vi "Configure.vi"(0 "Interface in":T5, 5 "Configuration":T1={"PLLgains"={"proportional gain"=0.0, "integral gain"=0.0}, "PLLrange"={"output high (Inf)"=inf, "output low (-Inf)"=-inf}, "dT"=0.0, "expectedFreq"=0.0, "lockDuration"=0.0, "freqBoundaries"=0.0, "adjustTheta"=0.0, "HarmonicFilter"={"enable"=FALSE, "coeff"={"ak"=0.0, "bk"=0.0}}} {"PLLgains"."proportional gain" step=0.125}, 11 "error in":errorcluster) -> (4 "Interface out":T5, 15 "error out":errorcluster)   [LabVIEW 2017, in "ThreePhasePLLInterface.lvlib"]
uses:
  ThreePhasePLLInterface.lvlib
  InterfaceRef.ctl
  <instrlib>/_niInstr/Instruction Framework/v1/Host/Instruction Target/niInstr Instruction Target v1 Host.lvclass
  <instrlib>/_niInstr/Instruction Framework/v1/Host/Instruction Framework Context/niInstr Instruction Framework Context v1 Host.lvclass
  Configuration.ctl
  <vilib>/rvi/Analysis/control/PID/Typedef/niFpgaPID_PIGains.ctl
  <vilib>/rvi/Analysis/control/PID/Typedef/niFpgaPID_OutputRange.ctl
  FPGA/HarmonicFilter.ctl
  FPGA/ThreePhasePLL.lvlib
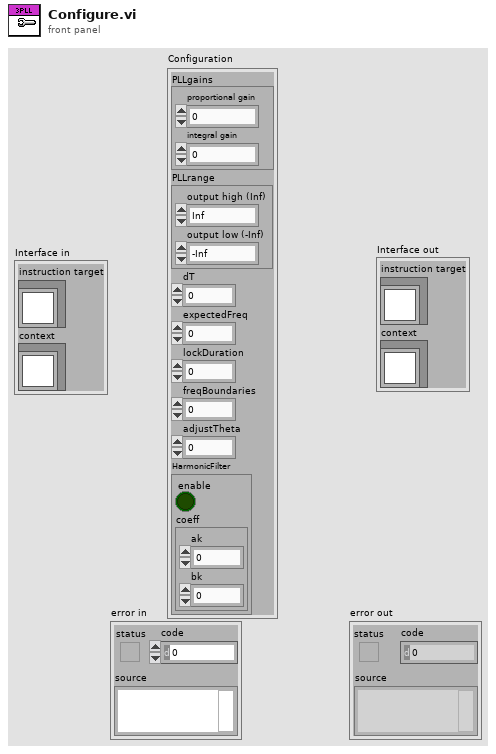
[diagram p1: front panel]
types:
  T1 = typedef "ThreePhasePLLInterface.lvlib/Configuration.ctl" = cluster{"PLLgains":T2, "PLLrange":T3, "dT":sgl, "expectedFreq":sgl, "lockDuration":sgl, "freqBoundaries":sgl, "adjustTheta":sgl, "HarmonicFilter":cluster{"enable":bool, "coeff":T4}}
  T2 = typedef "niFpgaPID_PIGains.ctl" = cluster{"proportional gain":sgl, "integral gain":sgl}
  T3 = typedef "niFpgaPID_OutputRange.ctl" = cluster{"output high (Inf)":sgl, "output low (-Inf)":sgl}
  T4 = typedef "ThreePhasePLL.lvlib/HarmonicFilter.ctl" = cluster{"ak":sgl, "bk":sgl}
  T5 = typedef "ThreePhasePLLInterface.lvlib/InterfaceRef.ctl" = cluster{"instruction target":refnum<class "niInstr Instruction Target v1 Host.lvclass">, "context":refnum<class "niInstr Instruction Framework Context v1 Host.lvclass">}
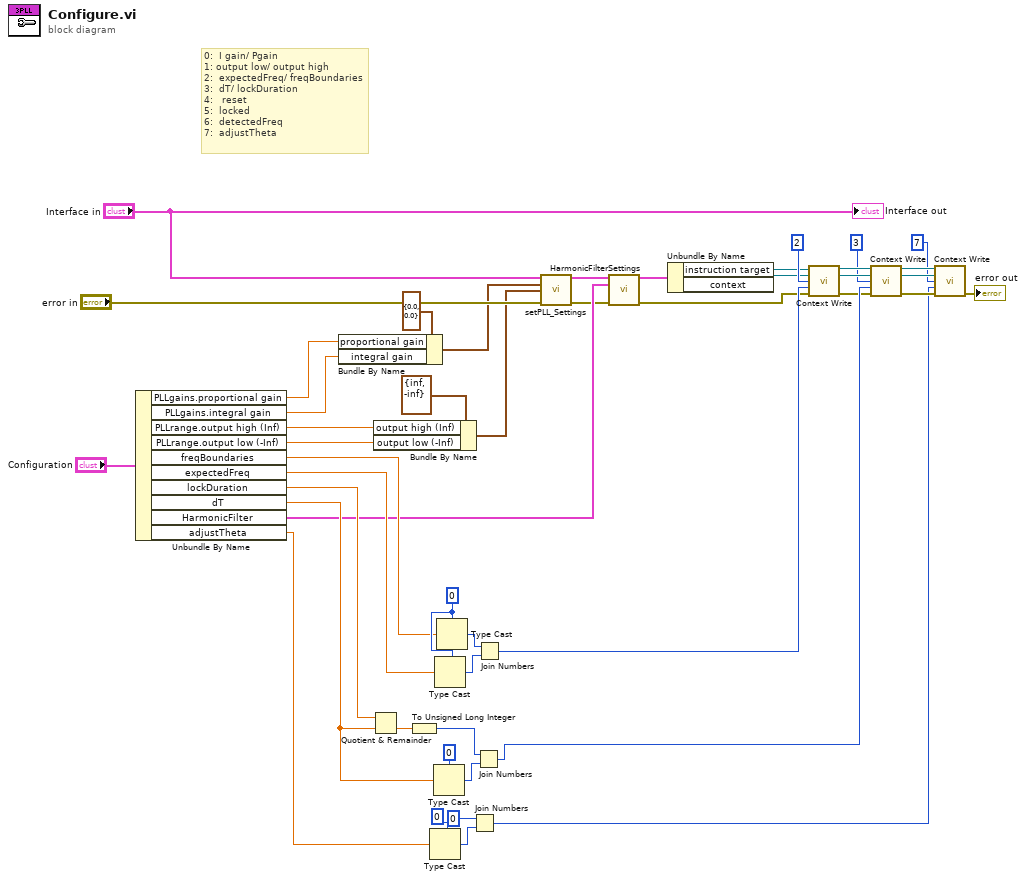
[diagram p0: block diagram]
diagram:
  w45 = u32 0
  # "0:  I gain/ Pgain\n1: output low/ output high\n2:  expectedFreq/ freqBoundaries\n3:  dT/ lockDuration\n4:   reset\n5:  locked\n6:  detectedFreq\n7:  adjustTheta"
  n1 = Unbundle By Name("Configuration") -> ("PLLgains.proportional gain"=w13:sgl, "PLLgains.integral gain"=w12:sgl, "PLLrange.output high (Inf)"=w9:sgl, "PLLrange.output low (-Inf)"=w8:sgl, "freqBoundaries"=w42:sgl, "expectedFreq"=w20:sgl, "lockDuration"=w23:sgl, "dT"=w19:sgl, "HarmonicFilter"=w4:cluster{"enable":bool, "coeff":T4}, "adjustTheta"=w1:sgl)
  n2 = Bundle By Name(cluster=T2 {"proportional gain"=0.0, "integral gain"=0.0} ("PLLgains"), "proportional gain"=w13, "integral gain"=w12) -> (w11:T2)
  n3 = Quotient & Remainder(x=w23, y=w19) -> (floor(x/y)=w22:sgl)  [unwired: 1 out]
  n4 = Bundle By Name(cluster=T3 {"output high (Inf)"=inf, "output low (-Inf)"=-inf} ("PLLrange"), "output high (Inf)"=w9, "output low (-Inf)"=w8) -> (w7:T3)
  n5 = To Unsigned Long Integer(number=w22) -> (unsigned 32bit integer=w21:u32)
  n6 = Type Cast(type=u32 0, x=w1) -> (*(type *) &x=w27:u32)
  n7 = Type Cast(type=u32 0, x=w19) -> (*(type *) &x=w39:u32)
  n8 = Type Cast(type=w45, x=w20) -> (*(type *) &x=w43:u32)
  n9 = Type Cast(type=w45, x=w42) -> (*(type *) &x=w44:u32)
  n10 = Join Numbers(hi=u32 0, lo=w27) -> ((hi.lo)=w25:u64)
  n11 = Join Numbers(hi=w21, lo=w39) -> ((hi.lo)=w34:u64)
  n12 = Join Numbers(hi=w44, lo=w43) -> ((hi.lo)=w40:u64)
  n13 = call "setPLL_Settings.vi"("Interface in"="Interface in", "PLLgains"=w11, "PLLrange"=w7, "error in"="error in") -> ("Interface out"=w6:T5, "error out"=w2:errorcluster)  [unwired: 10 in]
  n14 = call "HarmonicFilterSettings.vi"("Interface in"=w6, "HarmonicFilterSettings"=w4, "error in"=w2) -> ("Interface out"=w5:T5, "error out"=w3:errorcluster)  [unwired: 11 in]
  n15 = Unbundle By Name(w5) -> ("instruction target"=w18:refnum<class "niInstr Instruction Target v1 Host.lvclass">, "context"=w17:refnum<class "niInstr Instruction Framework Context v1 Host.lvclass">)
  n16 = call <instrlib>:"Context Write.vi"("instruction target in"=w18, "context in"=w17, "address"=u64 2, "data"=w40, "error in"=w3) -> ("instruction target out"=w37:refnum<class "niInstr Instruction Target v1 Host.lvclass">, "context out"=w36:refnum<class "niInstr Instruction Framework Context v1 Host.lvclass">, "error out"=w33:errorcluster)  [unwired: 8 in]
  n17 = call <instrlib>:"Context Write.vi"("instruction target in"=w37, "context in"=w36, "address"=u64 3, "data"=w34, "error in"=w33) -> ("instruction target out"=w32:refnum<class "niInstr Instruction Target v1 Host.lvclass">, "context out"=w30:refnum<class "niInstr Instruction Framework Context v1 Host.lvclass">, "error out"=w31:errorcluster)  [unwired: 8 in]
  n18 = call <instrlib>:"Context Write.vi"("instruction target in"=w32, "context in"=w30, "address"=u64 7, "data"=w25, "error in"=w31) -> ("error out"=→"error out":errorcluster)  [unwired: 8 in, 2 out]
  "Interface out" <- "Interface in"
